vi "PRODUCTION_YEAR_main.vi"() -> ()   [LabVIEW 2017]
uses:
  <vilib>/Math Plots/3D Math Plots/3D Pie/3D Pie XCtrl/3D Pie.xctl
  <vilib>/addons/database/Connection.llb/DB Tools Open Connec (Path).vi
  <vilib>/Math Plots/3D Math Plots/3D Pie/3D Pie Datatype/Public/Plot Helper (Vector).vi
  <vilib>/addons/database/NI_Database_API.lvlib
  <vilib>/Math Plots/3D Math Plots/3D Pie/3D Pie Datatype/3D Pie Datatype.lvclass
panel:
  in  "Tab Control":enum32{"Data", "Graph"}(tab)
  out "Table":string[][](table)=[["January", "0", "0", "0", "0", "0", "0", "0"], ["February", "0", "0", "0", "0", "0", "0", "0"], ["March", "0", "0", "0", "0", "0", "0", "0"], ["April", "0", "0", "0", "0", "0", "0", "0"], ["May", "0", "0", "0", "0", "0", "0", "0"], ["June", "0", "0", "0", "0", "0", "0", "0"], ["July", "0", "0", "0", "0", "0", "0", "0"], ["August", "0", "0", "0", "0", "0", "0", "0"], ["September", "0", "0", "0", "0", "0", "0", "0"], ["October", "0", "0", "0", "0", "0", "0", "0"], ["November", "0", "0", "0", "0", "0", "0", "0"], ["December", "0", "0", "0", "0", "0", "0", "0"]]
  out "3D Pie":refnum<class "3D Plot Datatype.lvclass">[](xcontrol)
  out "String":string="Processing...\nPlease wait!"
  out "All Days":string[](array[string])
  in  "Select Year":string(combo)
  in  "Select Month":string(combo)
  out "Station Count":i32
  out "All Shifts":bool
  in  "Cancel Button - Archive":bool
  in  "Download 2":bool
  in  "Get Rport 2":bool
  out "error out":errorcluster
  in  "error in (no error)":errorcluster
  in  "Shift":string(combo)
  in  "Station":string(combo)
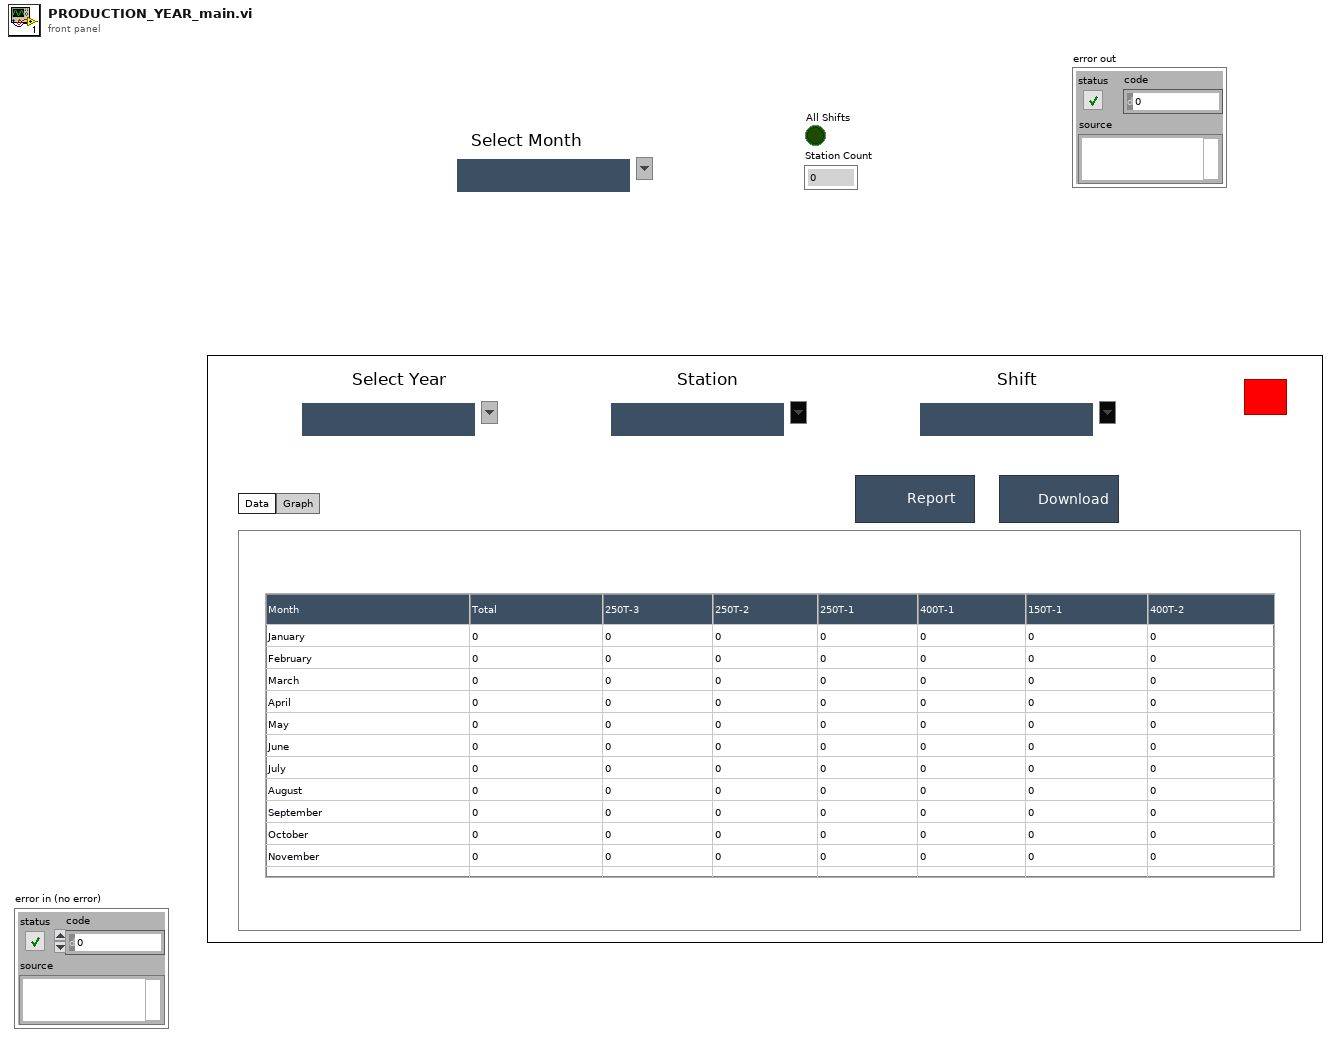
[diagram p1: front panel]
types:
  T1 = typedef "NI_Database_API.lvlib/Conn ObjectReference.ctl" = refnum<k1>
  T2 = enum32{"invalid app kind", "Development System", "Run Time System", "Student Edition", "Embedded LabVIEW", "Evaluation", "Custom"}
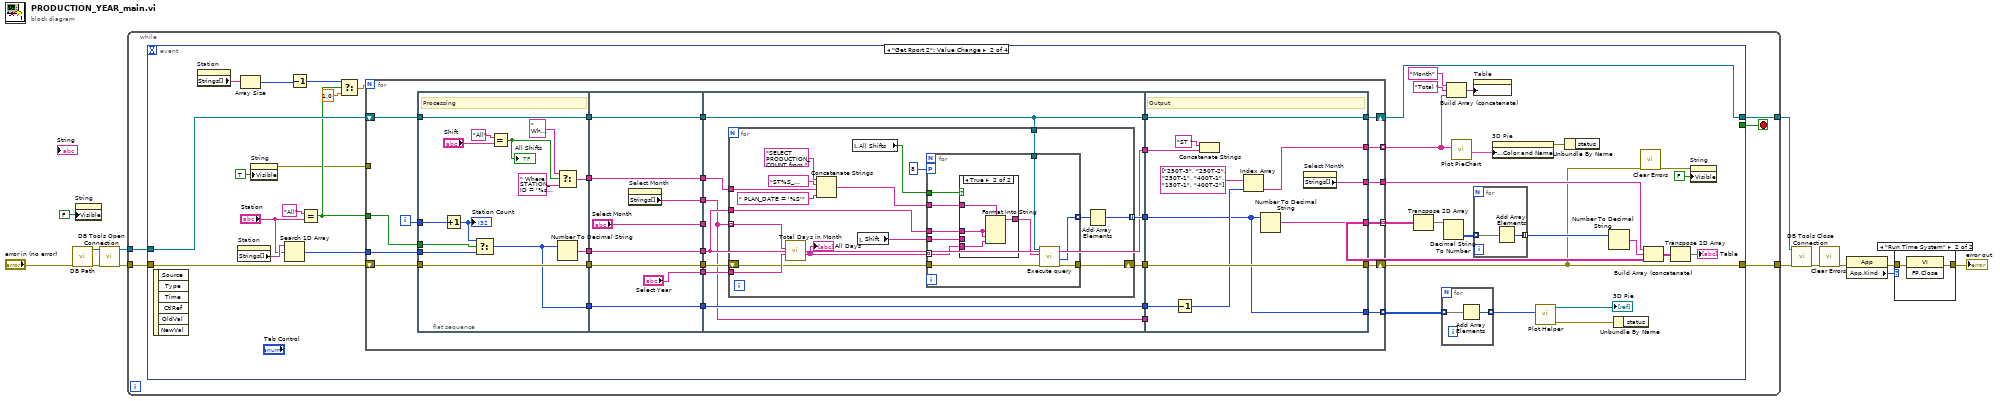
[diagram p0: block diagram]
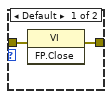
[diagram p2: hidden frame]
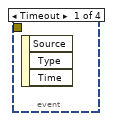
[diagram p3: hidden frame]
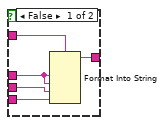
[diagram p4: hidden frame]
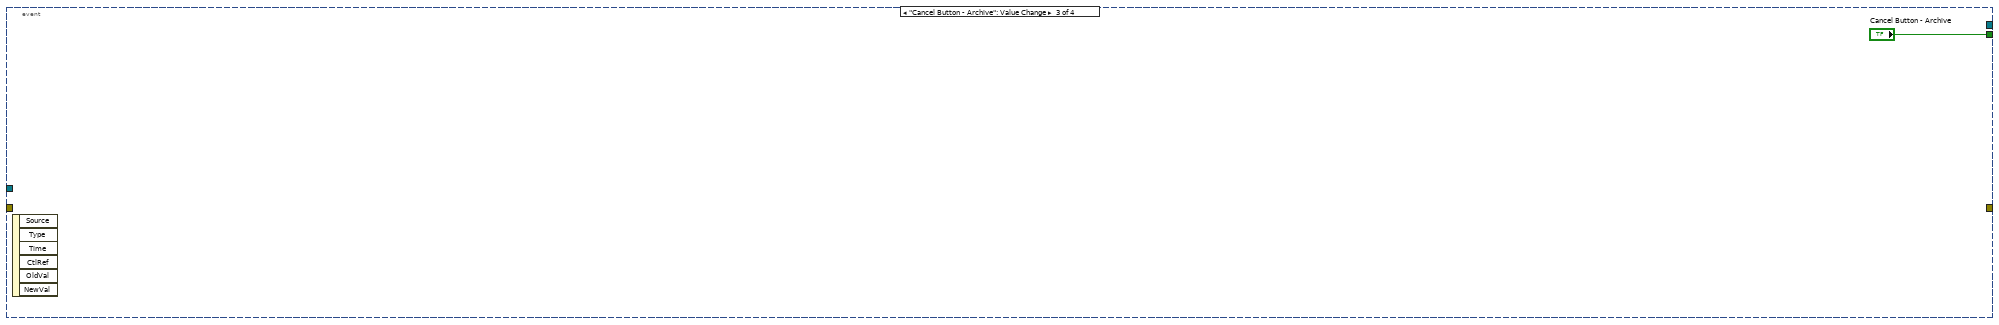
[diagram p5: hidden frame]
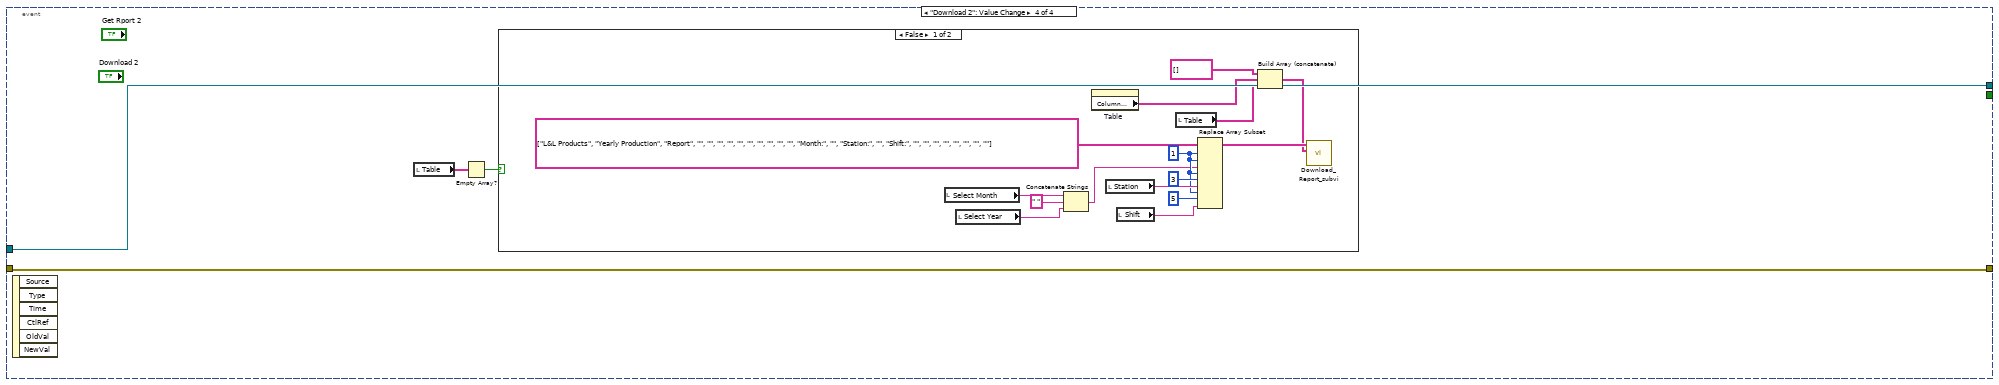
[diagram p6: hidden frame]
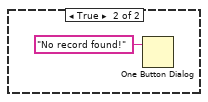
[diagram p7: hidden frame]
diagram:
  n1 = call "DB Path.vi"("error in"="error in (no error)") -> ("error out"=w13:errorcluster, "DB Path"=w12:path)  [unwired: 9 in]
  n2 = property on="String" class="Str"("Visible"=FALSE) -> ()  [unwired: 2 in, 2 out]
  n3 = call-poly <vilib>:"DB Tools Open Connection.vi"("error in (no error)"=w13, "connection information"=w12) -> ("error out"=w10:errorcluster, "connection reference"=w9:T1)  [unwired: 6 in]
  n4 = while {
    tunnel: w10 -> [w15]
    tunnel: w9 -> [w14]
    tunnel: [w17] -> w4
    tunnel: [w16] -> w3
    stop <- w18 stop-if-true
    n5 = event shown="[1] \"Get Rport 2\": Value Change" {
      selector: _ -> [_ _ _ _]
      dyn-events: _ -> [_ _ _ _]
      timeout: _ -> [_ _ _ _]
      tunnel: w14 -> [_ w54 _ w171]
      tunnel: [_ _ "Cancel Button - Archive" _] -> w18
      tunnel: [_ w30 _ w170] -> w17
      tunnel: [_ w53 _ w171] -> w16
      tunnel: w15 -> [_ w52 _ w170]
      event Timeout {
        n6 = event-data() -> ()  [unwired: 1 in, 3 out]
      }
      event "Get Rport 2": Value Change {
        n7 = event-data() -> ()  [unwired: 1 in, 6 out]
        n8 = property on="Station" class="CmbBox"() -> ("Strings[]"=w48:string[])  [unwired: 2 in, 2 out]
        n9 = property on="Station" class="CmbBox"() -> ("Strings[]"=w45:string[])  [unwired: 2 in, 2 out]
        n10 = Array Size(array=w48) -> (size(s)=w47:i32)
        n11 = property on="String" class="Str"("Visible"=TRUE) -> (error out=w28:errorcluster)  [unwired: 2 in, 1 out]
        n12 = Search 1D Array(1D array=w45, element="Station") -> (index of element=w42:i32)  [unwired: 1 in]
        n13 = Decrement(x=w47) -> (x-1=w46:i32)
        n14 = Equal?(x="All", y="Station") -> (x = y?=w43:bool)
        n15 = Select(t=w46, s=w43, f=1.0) -> (s? t:f=w50:dbl)
        n16 = for {
          N: w50 -> [_]
          shift-right: [w81] -> w53
          shift-left: w54 -> [w88]
          shift-right: [w82] -> w30
          shift-left: w52 -> [w87]
          tunnel: w43 -> [w86]
          tunnel: w42 -> [w85]
          tunnel: [w83] -> w21 mode=indexing
          tunnel: [w77] -> w35 mode=indexing
          tunnel: [w76] -> w38
          tunnel: w28 -> [_]
          tunnel: [w60] -> w20 mode=indexing
          i -> [w84]
          n17 = flat-sequence {
            tunnel: [w99] -> w74
            tunnel: [w100] -> w72
            tunnel: [w102] -> w70
            tunnel: [w101] -> w68
            tunnel: w84 -> [w94]
            tunnel: w85 -> [w95]
            tunnel: w86 -> [w96]
            tunnel: w87 -> [w99]
            tunnel: w88 -> [w100]
            tunnel: [w89] -> w61
            tunnel: w74 -> [w110]
            tunnel: [w110] -> w73
            tunnel: w72 -> [w109]
            tunnel: [w109] -> w71
            tunnel: w70 -> [w108]
            tunnel: [w108] -> w69
            tunnel: w68 -> [w107]
            tunnel: [w107] -> w67
            tunnel: ["Select Month"] -> w66
            tunnel: [w105] -> w65
            tunnel: ["Select Year"] -> w64
            tunnel: [w103] -> w62
            tunnel: w61 -> [w103]
            tunnel: w73 -> [w117]
            tunnel: [w116] -> w80
            tunnel: w71 -> [w118]
            tunnel: [w118] -> w79
            tunnel: w69 -> [w119]
            tunnel: w67 -> [w114]
            tunnel: [w115] -> w78
            tunnel: [w114] -> w75
            tunnel: w66 -> [_]
            tunnel: w65 -> [w111]
            tunnel: w64 -> [w113]
            tunnel: [w112] -> w63
            tunnel: w62 -> [w112]
            tunnel: [w111] -> w59
            tunnel: [w159] -> w83
            tunnel: w80 -> [w161]
            tunnel: [w161] -> w82
            tunnel: [w166] -> w81
            tunnel: w79 -> [w166]
            tunnel: w78 -> [w156]
            tunnel: [w165] -> w77
            tunnel: [w162] -> w76
            tunnel: w75 -> [w164]
            tunnel: w63 -> [w158]
            tunnel: [w156] -> w60
            tunnel: w59 -> [_]
            frame #0 {
              # "Processing"
              n18 = Increment(x=w94) -> (x+1=w93:i32)
              "Station Count" <- w93
              n19 = Select(t=w93, s=w96, f=w95) -> (s? t:f=w89:i32)
              n20 = Equal?(x="All", y="Shift") -> (x = y?=w92:bool)
              "All Shifts" <- w92
              n21 = Select(t=" Where STATION_ID = '%s' and " ("format string"), s=w92, f=" Where STATION_ID = '%s' and SHIFT = '%s' and" ("format string")) -> (s? t:f=w102:string)
              n22 = Number To Decimal String(number=w89) -> (decimal integer string=w101:string)  [unwired: 1 in]
            }
            frame #1 {
              n23 = property on="Select Month" class="CmbBox"() -> ("Strings[]"=w105:string[])  [unwired: 2 in, 2 out]
            }
            frame #2 {
              n24 = for {
                tunnel: w119 -> [w134]
                tunnel: w118 -> [w129]
                tunnel: [w123] -> w115 mode=indexing
                tunnel: w114 -> [w128]
                tunnel: w111 -> [w126] mode=indexing
                shift-right: [w121] -> w116
                shift-left: w117 -> [w122]
                tunnel: w113 -> [w125]
                n25 = call "Total Days in Month.vi"("Year"=w125, "Month"=w126) -> ("All Days"=w127:string[])  [unwired: 8 in, 1 out]
                "All Days" <- w127
                n26 = Concatenate Strings("SELECT  PRODUCTION_COUNT from " ("format string"), "ST%S_PRODUCTION_COUNT", w134, " PLAN_DATE = '%S'" ("string")) -> (w131:string)
                n27 = local read "All Shifts"() -> (w132:bool)
                n28 = local read "Shift"() -> (w130:string)
                n29 = for {
                  tunnel: w132 -> [w146]
                  tunnel: w131 -> [w145]
                  tunnel: w128 -> [w144]
                  tunnel: w130 -> [w143]
                  tunnel: w127 -> [w142] mode=indexing
                  tunnel: w129 -> [w140]
                  tunnel: [w139] -> w124 mode=indexing
                  workers-P: 8 -> [_]
                  tunnel: w122 -> [w138]
                  tunnel: [w137] -> w121
                  n30 = case shown="True" w146 {
                    tunnel: w145 -> [w151 w155]
                    tunnel: w144 -> [w150 w154]
                    tunnel: w143 -> [w149 _]
                    tunnel: w142 -> [w148 w153]
                    tunnel: [w147 w152] -> w141
                    frame False {
                      n31 = Format Into String(format string=w151, w150, w150, w149, w148) -> (resulting string=w147:string)  [unwired: 2 in, 1 out]
                    }
                    frame True {
                      n32 = Format Into String(format string=w155, w154, w154, w153) -> (resulting string=w152:string)  [unwired: 2 in, 1 out]
                    }
                  }
                  n33 = call "Execute query.vi"("error in (no error)"=w138, "String"=w141, "connection reference"=w140) -> ("error out"=w137:errorcluster, "Production Count"=w139:i32)  [unwired: 3 in, 4 out]
                }
                n34 = Add Array Elements(numeric array=w124) -> (sum=w123:i32)
              }
            }
            frame #3 {
              # "Output"
              n35 = Decrement(x=w158) -> (x-1=w157:i32)
              n36 = Concatenate Strings("ST " ("string"), w164) -> ()  [unwired: 1 out]
              n37 = Index Array(array=string[] ["250T-3", "250T-2", "250T-1", "400T-1", "150T-1", "400T-2"], index=w157) -> (element=w159:string)
              n38 = Number To Decimal String(number=w156) -> (decimal integer string=w165:string[])  [unwired: 1 in]
              n39 = property on="Select Month" class="CmbBox"() -> ("Strings[]"=w162:string[])  [unwired: 2 in, 2 out]
            }
          }
        }
        n40 = Transpose 2D Array(2D array=w35) -> (transposed array=w34:string[][])
        n41 = for {
          tunnel: w20 -> [w56] mode=indexing
          tunnel: [w55] -> w24 mode=indexing
          n42 = Add Array Elements(numeric array=w56) -> (sum=w55:i32)
        }
        n43 = Decimal String To Number(string=w34) -> (number=w33:i32[][])  [unwired: 2 in, 1 out]
        n44 = Build Array (concatenate)("Month", "Total ", w21) -> (w41:string[])
        n45 = call "Plot PieChart.vi"("Label"=w21) -> ("Labelling"=w22:cluster{dbl, "String":string}[])  [unwired: 10 in]
        n46 = property on="Table" class="Tbl (strict)"("Column Headers[]"=w41) -> ()  [unwired: 2 in, 2 out]
        n47 = for {
          tunnel: w33 -> [w58] mode=indexing
          tunnel: [w57] -> w32 mode=indexing
          n48 = Add Array Elements(numeric array=w58) -> (sum=w57:i32)
        }
        n49 = property on="3D Pie" class="3D Pie (strict)"("Plot Specific:Color and Name"=w22) -> (error out=w19:errorcluster)  [unwired: 2 in, 1 out]
        n50 = call-poly <vilib>:"Plot Helper.vi"("x vector"=w24) -> ("error out"=w25:errorcluster, "3D Plot lvclass Array out"=→"3D Pie":refnum<class "3D Plot Datatype.lvclass">[])  [unwired: 2 in, 7 out]
        n51 = Unbundle By Name(w19) -> ()  [unwired: 1 out]
        n52 = Number To Decimal String(number=w32) -> (decimal integer string=w31:string[])  [unwired: 1 in]
        n53 = Unbundle By Name(w25) -> ()  [unwired: 1 out]
        n54 = call <vilib>:"Clear Errors.vi"("error in (no error)"=w30) -> ("error out"=w26:errorcluster)  [unwired: 5 in, 1 out]
        n55 = Build Array (concatenate)(w38, w31, w35) -> (w40:string[][])
        n56 = Transpose 2D Array(2D array=w40) -> (transposed array=→"Table":string[][])
        n57 = property on="String" class="Str"(error in=w26, "Visible"=FALSE) -> ()  [unwired: 1 in, 2 out]
      }
      event "Cancel Button - Archive": Value Change {
        n58 = event-data() -> ()  [unwired: 1 in, 6 out]
      }
      event "Download 2": Value Change {
        n59 = event-data() -> ()  [unwired: 1 in, 6 out]
        n60 = local read "Table"() -> (w168:string[][])
        n61 = Empty Array?(array=w168) -> (empty?=w169:bool)
        n62 = case shown="False" w169 {
          frame False {
            w182 = 1 ("index (row)")
            n63 = local read "Select Month"() -> (w179:string)
            n64 = local read "Select Year"() -> (w178:string)
            n65 = Concatenate Strings(w179, " " ("string"), w178) -> (w177:string)
            n66 = property on="Table" class="Tbl (strict)"() -> ("Column Headers[]"=w172:string[])  [unwired: 2 in, 2 out]
            n67 = local read "Station"() -> (w183:string)
            n68 = local read "Shift"() -> (w180:string)
            n69 = local read "Table"() -> (w173:string[][])
            n70 = Replace Array Subset(array=string[][] [["L&L Products", "Yearly Production", "Report", "", "", "", "", "", "", "", "", "", ""], ["Month:", "", "Station:", "", "Shift:", "", "", "", "", "", "", "", ""]] ("Column Header Strings[]"), new element #1=w177, index (row) #1=w182, index (col) #1=w182, new element #2=w183, index (row) #2=w182, index (col) #2=3 ("disabled index (col)"), new element #3=w180, index (row) #3=w182, index (col) #3=5 ("disabled index (col)")) -> (w185:string[][])
            n71 = Build Array (concatenate)(string[] [] ("element"), w172, w173) -> (w174:string[][])
            n72 = call "Download_Report_subvi.vi"("Value"=w174, "Column Header Strings[]"=w185) -> ()  [unwired: 9 in, 1 out]
          }
          frame True {
            n73 = One Button Dialog(message="No record found!") -> ()  [unwired: 1 in, 1 out]
          }
        }
      }
    }
  }
  n74 = call <vilib>:"DB Tools Close Connection.vi"("error in (no error)"=w4, "connection reference"=w3) -> ("error out"=w6:errorcluster)  [unwired: 5 in]
  n75 = call <vilib>:"Clear Errors.vi"("error in (no error)"=w6) -> ("error out"=w5:errorcluster)  [unwired: 5 in, 1 out]
  n76 = property class="App"(error in=w5) -> (error out=w7:errorcluster, "App.Kind"=w8:T2)  [unwired: 1 in, 1 out]
  n77 = case shown="\"Run Time System\"" w8 {
    tunnel: w7 -> [w189 w191]
    tunnel: [w188 w190] -> w2
    frame Default {
      n78 = invoke class="VI" method="FP.Close"(error in=w189) -> (error out=w188:errorcluster)  [unwired: 2 in, 2 out]
    }
    frame "Run Time System" {
      n79 = invoke class="VI" method="FP.Close"(error in=w191) -> (error out=w190:errorcluster)  [unwired: 2 in, 2 out]
    }
  }
  "error out" <- w2
